vi "microspec_validating - Kopie.vi"() -> ()   [LabVIEW 2013]
uses:
  <vilib>/Instr/_visa.llb/VISA Configure Serial Port (Instr).vi
  <vilib>/Utility/file.llb/Write To Spreadsheet File (string).vi
panel:
  out "error 2":dbl
  in  "Path":path
  in  "intergration time":dbl=54.0 caption="sensor\nintergration time (us)" min=54.0 max=1000000.0 step=100.0
  in  "?":T1(tab)=enum."measuring sequence"
  out "radiometer data file path":path
  in  "Runname":string
  out "Sensor_name":string="ILT1400"
  out "Radiometer Average":dbl
  in  "Delay":dbl=1.0
  in  "Step":dbl=1.0
  in  "Stop Wl":dbl=900.0 min=0.0 max=5000.0 step=100.0
  in  "Start Wl":dbl=300.0 min=0.0 max=5000.0 step=100.0
  in  "mean_number":i32=1 caption="Mean Number"
  out "Current Wavelength":dbl
  out "XY-Graph 2":cluster{"Y":dbl[], "Y":dbl[]}[](graph)
  in  "run 5":bool
  out "sectrometer data file path":path
  in  "save data":bool
  in  "reset with every wavelength?":bool caption="reset with new run?"
  in  "Delay":dbl=1.0
  in  "Step":dbl=10.0
  in  "Stop Wl":dbl=900.0 min=0.0 max=5000.0 step=100.0
  out "Current Wavelength":dbl
  in  "Start Wl 2":dbl=300.0 min=0.0 max=5000.0 step=10.0
  in  "Sensor":string(combo)="C12880MA_15B00040"
  in  "run 2":bool
  in  "Set Runs":i32=1
  out "Current Run":i32
  in  "stop runs":bool
  out "raw_data":cluster{"Y":dbl[], "Y":dbl[]}[](graph) caption="raw data"
  out "error":dbl
  out "raw_data 2":cluster{"Y":dbl[], "Y":dbl[]}[](graph) caption="raw data"
  in  "Stopp":bool
  out "System Setup":i32
  out "DLL Version":string
  out "Get Version":i32
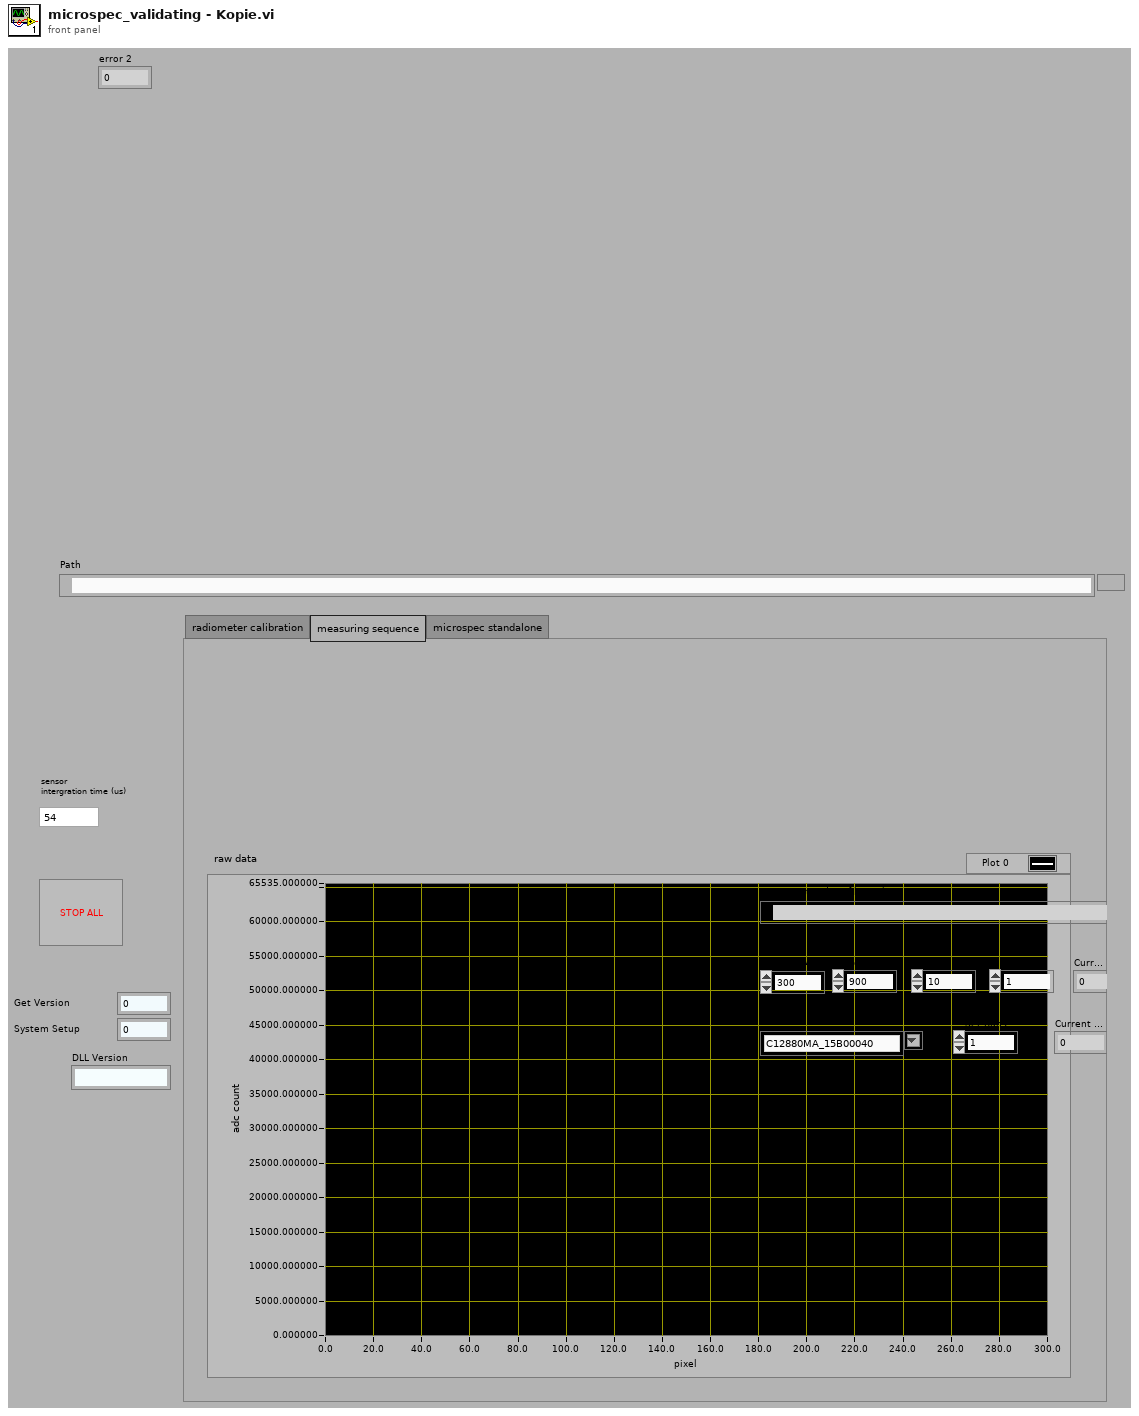
[diagram p1: front panel]
types:
  T1 = enum32{"radiometer calibration", "measuring sequence", "microspec standalone"}
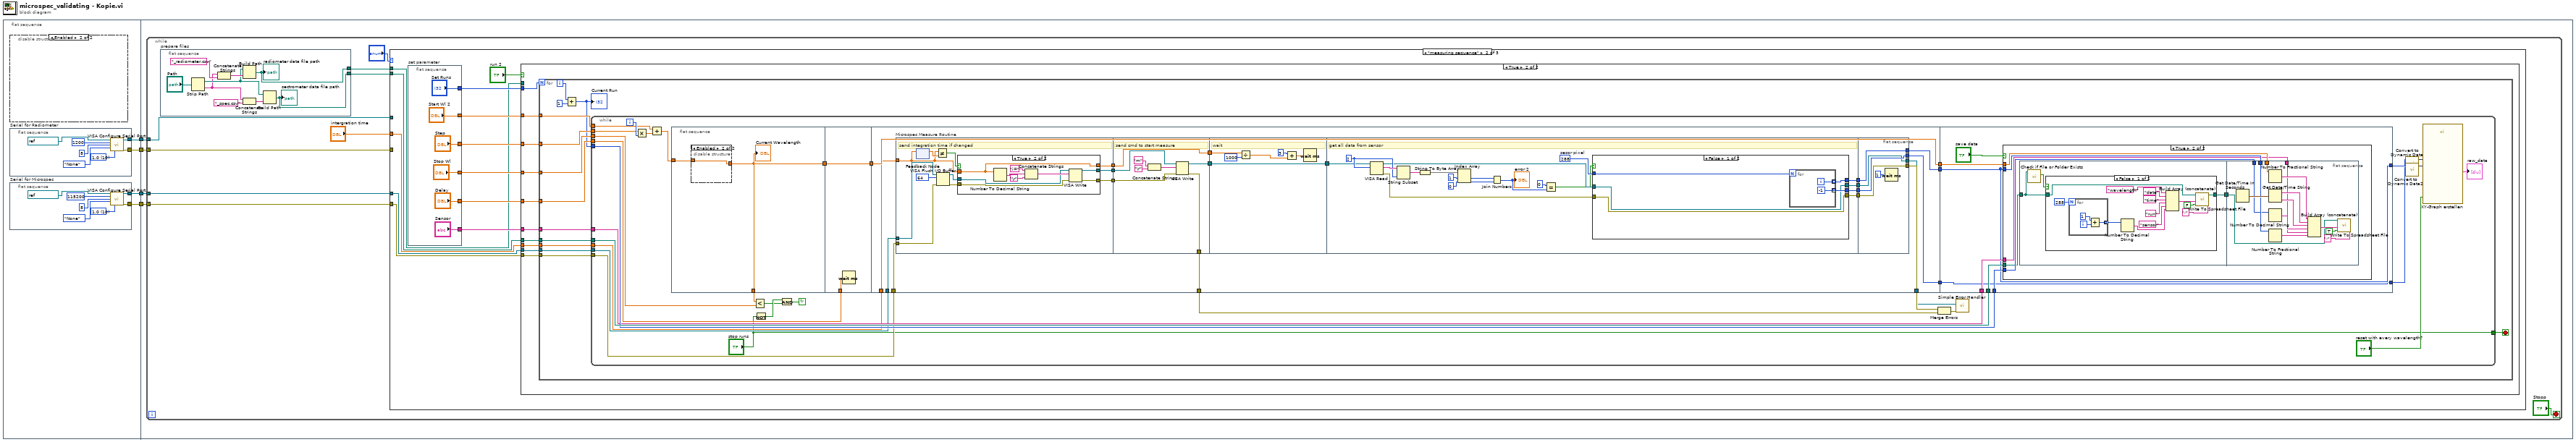
[diagram p0: block diagram]
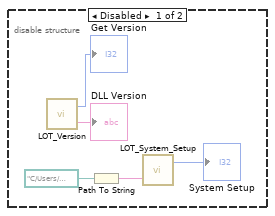
[diagram p2: hidden frame]
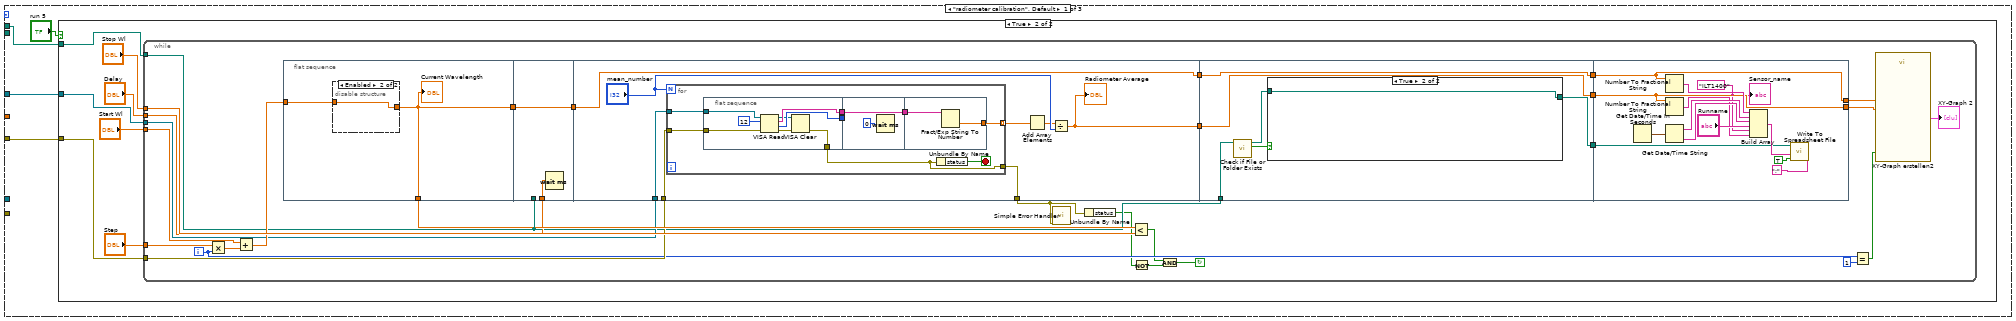
[diagram p3: hidden frame]
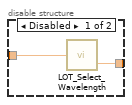
[diagram p5: hidden frame]
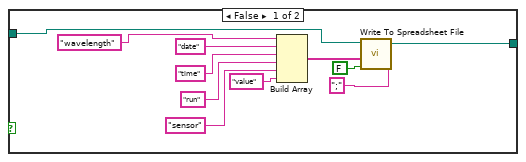
[diagram p6: hidden frame]
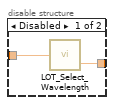
[diagram p8: hidden frame]
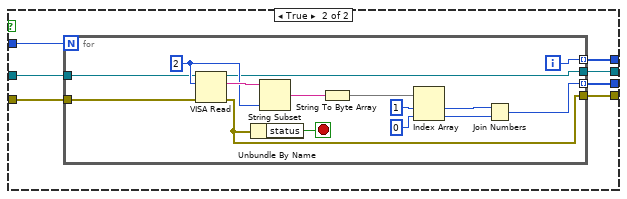
[diagram p10: hidden frame]
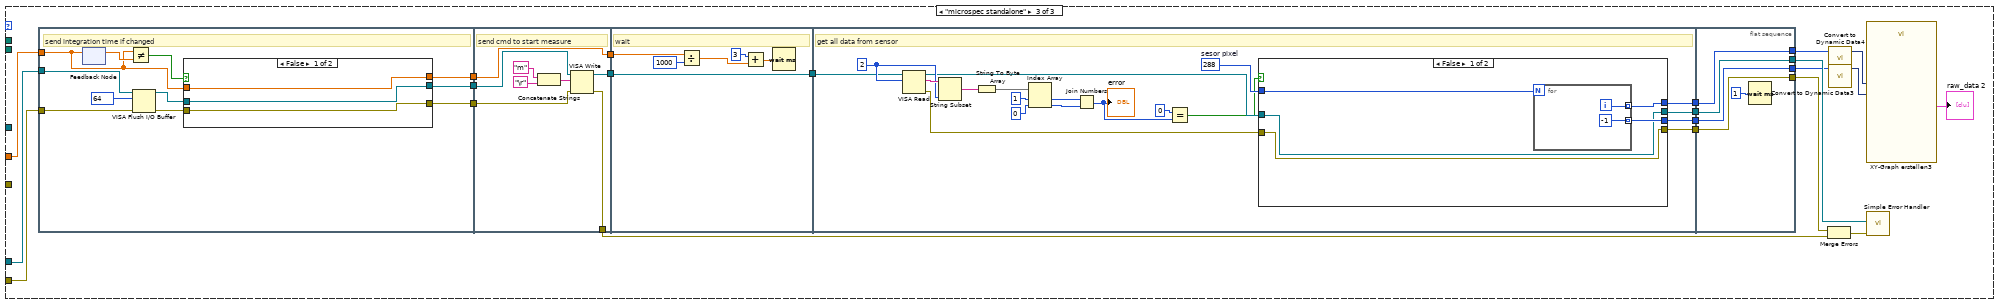
[diagram p13: hidden frame]
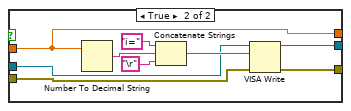
[diagram p14: hidden frame]
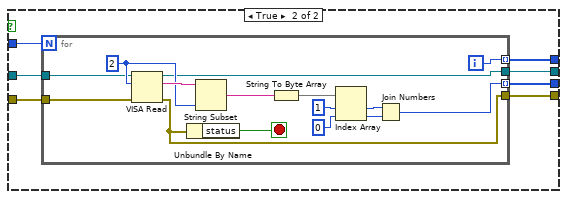
[diagram p15: hidden frame]
diagram:
  n1 = flat-sequence {
    tunnel: [w8] -> w4
    tunnel: [w7] -> w3
    tunnel: [w6] -> w2
    tunnel: [w5] -> w1
    tunnel: w4 -> [w31]
    tunnel: w3 -> [w30]
    tunnel: w2 -> [w29]
    tunnel: w1 -> [w28]
    frame #0 {
      # "Configuration"
      n2 = disable-structure shown="Enabled" {
        frame Disabled {
          n3 = call "LOT_Version.vi"() -> ("Version"=→"DLL Version":string, "Get Version"=→"Get Version":i32)
          n4 = Path To String(path=path "C:/Users/Public/Documents/LOT/Monochromator Control/Configurations/LOT_MSH-300_SN16578.xml" ("Configuration File")) -> (string=w25:string)
          n5 = call "LOT_System_Setup.vi"("CFG File Path"=w25) -> ("Error Code"=→"System Setup":i32)  [unwired: 2 in]
        }
        frame Enabled {
        }
      }
      n6 = flat-sequence "Serial for Radiometer" {
        tunnel: [w15] -> w6
        tunnel: [w14] -> w5
        frame #0 {
          w10 = u16 10 items=["1.0"=10, "1.5"=15, "2.0"=20] ("stop bits (10: 1 bit)")
          n7 = call-poly "VISA Configure Serial Port"("VISA resource name"=refnum<visa-resource-name> "COM4", "baud rate (9600)"=u32 1200, "data bits (8)"=u16 8, "parity (0:none)"=enum16{"None", "Odd", "Even", "Mark", "Space"}."None", "stop bits (10: 1 bit)"=w10) -> ("VISA resource name out"=w14:refnum<visa-resource-name>, "error out"=w15:errorcluster)  [unwired: 9 in]
        }
      }
      n8 = flat-sequence "Serial for Microspec" {
        tunnel: [w22] -> w8
        tunnel: [w21] -> w7
        frame #0 {
          w17 = u16 10 items=["1.0"=10, "1.5"=15, "2.0"=20] ("stop bits (10: 1 bit)")
          n9 = call-poly "VISA Configure Serial Port"("VISA resource name"=refnum<visa-resource-name> "COM11", "baud rate (9600)"=u32 115200, "data bits (8)"=u16 8, "parity (0:none)"=enum16{"None", "Odd", "Even", "Mark", "Space"}."None", "stop bits (10: 1 bit)"=w17) -> ("VISA resource name out"=w22:refnum<visa-resource-name>, "error out"=w21:errorcluster)  [unwired: 9 in]
        }
      }
    }
    frame #1 {
      n10 = while {
        tunnel: w31 -> [w38]
        tunnel: w30 -> [w37]
        tunnel: w29 -> [w36]
        tunnel: w28 -> [w35]
        stop <- "Stopp" stop-if-true
        n11 = flat-sequence "prepare files" {
          tunnel: [w41] -> w32
          tunnel: [w42] -> w33
          frame #0 {
            n12 = Strip Path(path="Path") -> (stripped path=w44:path, name=w43:string)
            n13 = Concatenate Strings(w43, "_radiometer.csv") -> (w45:string)
            n14 = Build Path(base path=w44, name or relative path=w45) -> (appended path=w42:path)
            "radiometer data file path" <- w42
            n15 = Concatenate Strings(w43, "_spec.csv") -> (w47:string)
            n16 = Build Path(base path=w44, name or relative path=w47) -> (appended path=w41:path)
            "sectrometer data file path" <- w41
          }
        }
        n17 = case shown="\"measuring sequence\"" "?" {
          tunnel: w32 -> [_ w165 _]
          tunnel: w38 -> [_ w164 w413]
          tunnel: w37 -> [_ w163 w412]
          tunnel: w36 -> [w52 _ _]
          tunnel: w35 -> [w51 _ _]
          tunnel: "intergration time" -> [_ w162 w411]
          tunnel: w33 -> [w50 w155 _]
          frame "radiometer calibration", Default {
            n18 = case shown="True" "run 5" {
              tunnel: w50 -> [_ w56]
              tunnel: w52 -> [_ w55]
              tunnel: w51 -> [_ w54]
              frame False {
              }
              frame True {
                n19 = while {
                  tunnel: "Step" -> [w88]
                  tunnel: "Start Wl" -> [w86]
                  tunnel: "Stop Wl" -> [w85]
                  tunnel: "Delay" -> [w81]
                  tunnel: w56 -> [w67]
                  tunnel: w54 -> [w80]
                  tunnel: w55 -> [w79]
                  i -> [w75]
                  stop <- w62 continue-if-true
                  n20 = Multiply(x=w88, y=w75) -> (x*y=w87:dbl)
                  n21 = Add(x=w86, y=w87) -> (x+y=w84:dbl)
                  n22 = flat-sequence {
                    tunnel: w84 -> [w90]
                    tunnel: [w89] -> w83
                    tunnel: [w89] -> w82
                    tunnel: w67 -> [_]
                    tunnel: w82 -> [w94]
                    tunnel: w81 -> [w95]
                    tunnel: [w94] -> w78
                    tunnel: w80 -> [w103]
                    tunnel: w79 -> [w102]
                    tunnel: w78 -> [w101]
                    tunnel: [w101] -> w71
                    tunnel: [w99] -> w69
                    tunnel: [w96] -> w61
                    tunnel: w71 -> [w129]
                    tunnel: [w129] -> w70
                    tunnel: w69 -> [w128]
                    tunnel: [w128] -> w68
                    tunnel: w67 -> [w126]
                    tunnel: [w127] -> w66
                    tunnel: [w145] -> w72
                    tunnel: [w146] -> w76
                    tunnel: w70 -> [w146]
                    tunnel: w68 -> [w145]
                    tunnel: w66 -> [w148]
                    frame #0 {
                      n23 = disable-structure shown="Enabled" {
                        disable-tunnel: w90 -> [w92 w93]
                        disable-tunnel: [w91 w93] -> w89
                        frame Disabled {
                          n24 = call "LOT_Select_Wavelength.vi"("Input Wavelength"=w92) -> ("Current Wavelength"=w91:dbl)  [unwired: 1 out]
                        }
                        frame Enabled {
                        }
                      }
                      "Current Wavelength" <- w89
                    }
                    frame #1 {
                      n25 = Wait (ms)(milliseconds to wait=w95) -> ()  [unwired: 1 out]
                    }
                    frame #2 {
                      n26 = for {
                        N: "mean_number" -> [_]
                        tunnel: w103 -> [w108]
                        tunnel: w102 -> [w107]
                        tunnel: [w106] -> w97 mode=indexing
                        tunnel: [w105] -> w96
                        stop <- w104 stop-if-true
                        n27 = flat-sequence {
                          tunnel: [w116] -> w111
                          tunnel: w108 -> [w119]
                          tunnel: w107 -> [w118]
                          tunnel: [w115] -> w110
                          tunnel: [w112] -> w105
                          tunnel: w111 -> [w121]
                          tunnel: [w121] -> w109
                          tunnel: w110 -> [_]
                          tunnel: w109 -> [w122]
                          tunnel: [w123] -> w106
                          frame #0 {
                            n28 = VISA Read(VISA resource name=w119, byte count=12, error in (no error)=w118) -> (VISA resource name out=w113:refnum<visa-resource-name>, read buffer=w116:string, return count=w115:u32, error out=w114:errorcluster)
                            n29 = VISA Clear(VISA resource name=w113, error in (no error)=w114) -> (error out=w112:errorcluster)  [unwired: 1 out]
                          }
                          frame #1 {
                            n30 = Wait (ms)(milliseconds to wait=u32 0 ("Zu wartende ms")) -> ()  [unwired: 1 out]
                          }
                          frame #2 {
                            n31 = Fract/Exp String To Number(string=w122) -> (number=w123:dbl)  [unwired: 3 in, 1 out]
                          }
                        }
                        n32 = Unbundle By Name(w105) -> ("status"=w104:bool)
                      }
                      n33 = Add Array Elements(numeric array=w97) -> (sum=w98:dbl)
                      n34 = Divide(x=w98, y="mean_number") -> (x/y=w99:dbl)
                      "Radiometer Average" <- w99
                    }
                    frame #3 {
                      n35 = call <vilib>:"Check if File or Folder Exists.vi"("path"=w126) -> ("file or folder exists?"=w125:bool, "dup path"=w124:path)  [unwired: 8 in, 1 out]
                      n36 = case shown="True" w125 {
                        tunnel: w124 -> [w138 w141]
                        tunnel: [w131 w141] -> w127
                        frame False {
                          n37 = Build Array("wavelength", "date" ("Element"), "time" ("Element"), "run" ("Element"), "sensor" ("Element"), "value") -> (w140:string[])
                          n38 = call-poly <vilib>:"Write To Spreadsheet File.vi"("delimiter (\\t)"=";", "append to file? (new file:F)"=FALSE, "1D data"=w140, "file path (dialog if empty)"=w138) -> ("new file path (Not A Path if cancelled)"=w131:path)  [unwired: 4 in]
                        }
                        frame True {
                        }
                      }
                    }
                    frame #4 {
                      w143 = "ILT1400" ("Sensor_name")
                      n39 = Get Date/Time In Seconds() -> (seconds since 1Jan1904=w153:timestamp)
                      n40 = Number To Fractional String(number=w146) -> (F-format string=w154:string)  [unwired: 3 in]
                      n41 = Number To Fractional String(number=w145) -> (F-format string=w142:string)  [unwired: 3 in]
                      n42 = Get Date/Time String(seconds (now)=w153) -> (date string=w152:string, time string=w151:string)  [unwired: 2 in]
                      n43 = Build Array(w154, w152, w151, "Runname", w143, w142) -> (w150:string[])
                      n44 = call-poly <vilib>:"Write To Spreadsheet File.vi"("delimiter (\\t)"=";", "append to file? (new file:F)"=TRUE, "1D data"=w150, "file path (dialog if empty)"=w148) -> ()  [unwired: 4 in, 1 out]
                      "Sensor_name" <- w143
                    }
                  }
                  n45 = call <vilib>:"Simple Error Handler.vi"("error in (no error)"=w61) -> ()  [unwired: 4 in, 5 out]
                  n46 = Unbundle By Name(w61) -> ("status"=w63:bool)
                  n47 = Less?(x=w83, y=w85) -> (x < y?=w65:bool)
                  n48 = Not(x=w63) -> (.not. x?=w64:bool)
                  n49 = And(x=w65, y=w64) -> (x .and. y?=w62:bool)
                  n50 = Equal?(x=w75, y=1) -> (x = y?=w73:bool)
                  n51 = call "XY-Graph erstellen2"("Reset"=w73, "Y Input"=w72, "X Input"=w76) -> ("XY Graph"=→"XY-Graph 2":cluster{"Y":dbl[], "Y":dbl[]}[])  [unwired: 7 in, 1 out]
                }
              }
            }
          }
          frame "measuring sequence" {
            n52 = flat-sequence "set parameter" {
              tunnel: ["Sensor"] -> w161
              tunnel: ["Delay"] -> w160
              tunnel: ["Step"] -> w159
              tunnel: ["Stop Wl"] -> w158
              tunnel: ["Start Wl 2"] -> w157
              tunnel: ["Set Runs"] -> w156
              frame #0 {
              }
            }
            n53 = case shown="True" "run 2" {
              tunnel: w165 -> [_ w173]
              tunnel: w161 -> [_ w182]
              tunnel: w156 -> [_ w181]
              tunnel: w164 -> [_ w180]
              tunnel: w163 -> [_ w179]
              tunnel: w160 -> [_ w178]
              tunnel: w158 -> [_ w177]
              tunnel: w159 -> [_ w176]
              tunnel: w157 -> [_ w175]
              tunnel: w162 -> [_ w174]
              tunnel: w155 -> [_ _]
              frame False {
              }
              frame True {
                n54 = for {
                  N: w181 -> [_]
                  tunnel: w173 -> [w195]
                  tunnel: w182 -> [w194]
                  tunnel: w180 -> [w193]
                  tunnel: w179 -> [w192]
                  tunnel: w178 -> [w191]
                  tunnel: w177 -> [w190]
                  tunnel: w176 -> [w189]
                  tunnel: w175 -> [w188]
                  tunnel: w174 -> [w187]
                  i -> [w186]
                  stop <- w183 stop-if-true
                  n55 = Add(x=w186, y=1) -> (x+y=w185:i32)
                  "Current Run" <- w185
                  n56 = while {
                    tunnel: w195 -> [w226]
                    tunnel: w185 -> [w225]
                    tunnel: w194 -> [w221]
                    tunnel: w193 -> [w219]
                    tunnel: w192 -> [w218]
                    tunnel: w191 -> [w209]
                    tunnel: w190 -> [w207]
                    tunnel: w189 -> [w206]
                    tunnel: w188 -> [w205]
                    tunnel: w187 -> [w204]
                    tunnel: ["stop runs"] -> w183
                    i -> [w223]
                    stop <- w198 continue-if-true
                    n57 = Multiply(x=w206, y=w223) -> (x*y=w228:dbl)
                    n58 = Add(x=w205, y=w228) -> (x+y=w227:dbl)
                    n59 = flat-sequence {
                      tunnel: w227 -> [w230]
                      tunnel: [w229] -> w224
                      tunnel: [w229] -> w208
                      tunnel: w224 -> [w234]
                      tunnel: w209 -> [w235]
                      tunnel: [w234] -> w212
                      tunnel: [w243] -> w220
                      tunnel: w219 -> [w247]
                      tunnel: w218 -> [w248]
                      tunnel: [w246] -> w216
                      tunnel: [w245] -> w215
                      tunnel: [w244] -> w214
                      tunnel: w212 -> [w243]
                      tunnel: w204 -> [w242]
                      tunnel: [w241] -> w203
                      tunnel: [w240] -> w196
                      tunnel: w226 -> [w351]
                      tunnel: w220 -> [w350]
                      tunnel: w225 -> [w349]
                      tunnel: [w347] -> w210
                      tunnel: w221 -> [w348]
                      tunnel: w214 -> [w347]
                      tunnel: w203 -> [w346]
                      tunnel: [w346] -> w202
                      frame #0 {
                        # "set wavelength"
                        n60 = disable-structure shown="Enabled" {
                          disable-tunnel: w230 -> [w232 w233]
                          disable-tunnel: [w231 w233] -> w229
                          frame Disabled {
                            n61 = call "LOT_Select_Wavelength.vi"("Input Wavelength"=w232) -> ("Current Wavelength"=w231:dbl)  [unwired: 1 out]
                          }
                          frame Enabled {
                          }
                        }
                        "Current Wavelength" <- w229
                      }
                      frame #1 {
                        # "wait"
                        n62 = Wait (ms)(milliseconds to wait=w235) -> ()  [unwired: 1 out]
                      }
                      frame #2 {
                        n63 = flat-sequence "Microspec Measure Routine" {
                          tunnel: w247 -> [w256]
                          tunnel: w248 -> [w265]
                          tunnel: [w260] -> w254
                          tunnel: [w259] -> w253
                          tunnel: [w258] -> w252
                          tunnel: w242 -> [w255]
                          tunnel: [w282] -> w251
                          tunnel: [w281] -> w245
                          tunnel: w254 -> [w279]
                          tunnel: w253 -> [w280]
                          tunnel: w252 -> [w278]
                          tunnel: [w278] -> w250
                          tunnel: w251 -> [w287]
                          tunnel: [w287] -> w249
                          tunnel: w250 -> [w286]
                          tunnel: w249 -> [w296]
                          tunnel: [w295] -> w239
                          tunnel: [w294] -> w238
                          tunnel: [w293] -> w237
                          tunnel: [w292] -> w236
                          tunnel: [w341] -> w240
                          tunnel: [w342] -> w246
                          tunnel: [w343] -> w241
                          tunnel: [w344] -> w244
                          tunnel: w239 -> [w344]
                          tunnel: w238 -> [w343]
                          tunnel: w237 -> [w342]
                          tunnel: w236 -> [w341]
                          frame #0 {
                            # "send integration time if changed"
                            n64 = feedback #1() -> (w264:dbl)  [unwired: 1 in]
                            n65 = feedback-in #1(w255) -> ()
                            n66 = Not Equal?(x=w255, y=w264) -> (x != y?=w263:bool)
                            n67 = VISA Flush I/O Buffer(VISA resource name=w256, mask (16)=64, error in (no error)=w265) -> (VISA resource name out=w262:refnum<visa-resource-name>, error out=w261:errorcluster)
                            n68 = case shown="True" w263 {
                              tunnel: w262 -> [w267 w273]
                              tunnel: w261 -> [w266 w272]
                              tunnel: [w266 w271] -> w260
                              tunnel: [w267 w270] -> w259
                              tunnel: w255 -> [w268 w269]
                              tunnel: [w268 w269] -> w258
                              frame False {
                              }
                              frame True {
                                n69 = Number To Decimal String(number=w269) -> (decimal integer string=w276:string)  [unwired: 1 in]
                                n70 = Concatenate Strings("i=", w276, "\r") -> (w274:string)
                                n71 = VISA Write(VISA resource name=w273, write buffer=w274, error in (no error)=w272) -> (VISA resource name out=w270:refnum<visa-resource-name>, error out=w271:errorcluster)  [unwired: 1 out]
                              }
                            }
                          }
                          frame #1 {
                            # "send cmd to start measure"
                            n72 = Concatenate Strings("m", "\r") -> (w283:string)
                            n73 = VISA Write(VISA resource name=w280, write buffer=w283, error in (no error)=w279) -> (VISA resource name out=w282:refnum<visa-resource-name>, error out=w281:errorcluster)  [unwired: 1 out]
                          }
                          frame #2 {
                            # "wait"
                            n74 = Divide(x=w286, y=u32 1000 ("Zu wartende ms")) -> (x/y=w288:dbl)
                            n75 = Add(x=u32 3 ("Zu wartende ms"), y=w288) -> (x+y=w290:dbl)
                            n76 = Wait (ms)(milliseconds to wait=w290) -> ()  [unwired: 1 out]
                          }
                          frame #3 {
                            w308 = 2
                            w310 = 288  # sesor pixel
                            # "get all data from sensor"
                            n77 = VISA Read(VISA resource name=w296, byte count=w308) -> (VISA resource name out=w301:refnum<visa-resource-name>, read buffer=w309:string, error out=w298:errorcluster)  [unwired: 1 in, 1 out]
                            n78 = String Subset(string=w309, length (rest)=w308) -> (substring=w307:string)  [unwired: 1 in]
                            n79 = String To Byte Array(string=w307) -> (unsigned byte array=w306:u8[])
                            n80 = Index Array(array=w306, index #1=1, index #2=0) -> (element #1=w302:u8, element #2=w303:u8)
                            n81 = Join Numbers(hi=w302, lo=w303) -> ((hi.lo)=w299:u16)
                            "error 2" <- w299
                            n82 = Equal?(x=0, y=w299) -> (x = y?=w297:bool)
                            n83 = case shown="False" w297 {
                              tunnel: [w313 w324] -> w293
                              tunnel: w301 -> [w312 w323]
                              tunnel: [w314 w322] -> w294
                              tunnel: [w315 w321] -> w295
                              tunnel: w310 -> [w311 w320]
                              tunnel: [w312 w319] -> w292
                              tunnel: w298 -> [w313 w318]
                              frame False {
                                n84 = for {
                                N: w311 -> [_]
                                tunnel: [-1] -> w314 mode=indexing
                                tunnel: [w317] -> w315 mode=indexing
                                i -> [w317]
                                }
                              }
                              frame True {
                                n85 = for {
                                N: w320 -> [_]
                                tunnel: w323 -> [w329]
                                tunnel: [w328] -> w324
                                tunnel: [w331] -> w322 mode=indexing
                                tunnel: [w330] -> w321 mode=indexing
                                tunnel: [w326] -> w319
                                tunnel: w318 -> [w325]
                                i -> [w330]
                                stop <- w327 stop-if-true
                                w338 = 2
                                n86 = VISA Read(VISA resource name=w329, byte count=w338, error in (no error)=w325) -> (VISA resource name out=w326:refnum<visa-resource-name>, read buffer=w339:string, error out=w328:errorcluster)  [unwired: 1 out]
                                n87 = Unbundle By Name(w328) -> ("status"=w327:bool)
                                n88 = String Subset(string=w339, length (rest)=w338) -> (substring=w337:string)  [unwired: 1 in]
                                n89 = String To Byte Array(string=w337) -> (unsigned byte array=w336:u8[])
                                n90 = Index Array(array=w336, index #1=1, index #2=0) -> (element #1=w332:u8, element #2=w333:u8)
                                n91 = Join Numbers(hi=w332, lo=w333) -> ((hi.lo)=w331:u16)
                                }
                              }
                            }
                          }
                          frame #4 {
                            n92 = Wait (ms)(milliseconds to wait=1) -> ()  [unwired: 1 out]
                          }
                        }
                      }
                      frame #3 {
                        n93 = case shown="True" "save data" {
                          tunnel: w351 -> [_ w354]
                          tunnel: w350 -> [_ w356]
                          tunnel: w349 -> [_ w355]
                          tunnel: w347 -> [_ w357]
                          tunnel: w348 -> [_ w353]
                          frame False {
                          }
                          frame True {
                            n94 = flat-sequence {
                              tunnel: w354 -> [w360]
                              tunnel: [w358] -> w352
                              tunnel: w357 -> [w384]
                              tunnel: w356 -> [w383]
                              tunnel: w355 -> [w382]
                              tunnel: w353 -> [w380]
                              tunnel: w352 -> [w378]
                              frame #0 {
                                n95 = call <vilib>:"Check if File or Folder Exists.vi"("path"=w360) -> ("file or folder exists?"=w359:bool)  [unwired: 8 in, 2 out]
                                n96 = case shown="False" w359 {
                                tunnel: w360 -> [w364 w377]
                                tunnel: [w361 w377] -> w358
                                frame False {
                                n97 = for {
                                N: 288 -> [_]
                                tunnel: [w374] -> w367 mode=indexing
                                i -> [w376]
                                n98 = Add(x=1, y=w376) -> (x+y=w374:i32)
                                }
                                n99 = Number To Decimal String(number=w367) -> (decimal integer string=w369:string[])  [unwired: 1 in]
                                n100 = Build Array (concatenate)("wavelength", "date" ("Element"), "time" ("Element"), "run" ("Element"), "sensor" ("Element"), w369) -> (w373:string[])
                                n101 = call-poly <vilib>:"Write To Spreadsheet File.vi"("delimiter (\\t)"=";", "append to file? (new file:F)"=FALSE, "1D data"=w373, "file path (dialog if empty)"=w364) -> ("new file path (Not A Path if cancelled)"=w361:path)  [unwired: 4 in]
                                }
                                frame True {
                                }
                                }
                              }
                              frame #1 {
                                n102 = Get Date/Time In Seconds() -> (seconds since 1Jan1904=w386:timestamp)
                                n103 = Number To Fractional String(number=w383) -> (F-format string=w385:string)  [unwired: 3 in]
                                n104 = Get Date/Time String(seconds (now)=w386) -> (date string=w387:string, time string=w388:string)  [unwired: 2 in]
                                n105 = Number To Decimal String(number=w382) -> (decimal integer string=w381:string)  [unwired: 1 in]
                                n106 = Number To Fractional String(number=w384) -> (F-format string=w391:string[])  [unwired: 3 in]
                                n107 = Build Array (concatenate)(w385, w387, w388, w381, w380, w391) -> (w389:string[])
                                n108 = call-poly <vilib>:"Write To Spreadsheet File.vi"("delimiter (\\t)"=";", "append to file? (new file:F)"=TRUE, "1D data"=w389, "file path (dialog if empty)"=w378) -> ()  [unwired: 4 in, 1 out]
                              }
                            }
                          }
                        }
                      }
                    }
                    n109 = Less?(x=w208, y=w207) -> (x < y?=w199:bool)
                    n110 = Not(x="stop runs") -> (.not. x?=w200:bool)
                    n111 = And(x=w200, y=w199) -> (x .and. y?=w198:bool)
                    n112 = Merge Errors(w216, w215) -> (w217:errorcluster)
                    n113 = call <vilib>:"Simple Error Handler.vi"("error source (\" \")"=w196, "error in (no error)"=w217) -> ()  [unwired: 3 in, 5 out]
                    n114 = call "Convert to Dynamic Data"("Array"=w202) -> ("Dynamic Data Type"=w211:dynamicdata)  [unwired: 3 in]
                    n115 = call "Convert to Dynamic Data2"("Array"=w210) -> ("Dynamic Data Type"=w213:dynamicdata)  [unwired: 3 in]
                    n116 = call "XY-Graph erstellen"("Reset"="reset with every wavelength?", "Y Input"=w213, "X Input"=w211) -> ("XY Graph"=→"raw_data":cluster{"Y":dbl[], "Y":dbl[]}[])  [unwired: 7 in, 1 out]
                  }
                }
              }
            }
          }
          frame "microspec standalone" {
            n117 = flat-sequence {
              tunnel: w413 -> [w423]
              tunnel: w412 -> [w424]
              tunnel: [w418] -> w410
              tunnel: [w417] -> w409
              tunnel: [w416] -> w408
              tunnel: w411 -> [w414]
              tunnel: [w441] -> w407
              tunnel: [w440] -> w403
              tunnel: w410 -> [w438]
              tunnel: w409 -> [w439]
              tunnel: w408 -> [w437]
              tunnel: [w437] -> w406
              tunnel: w407 -> [w446]
              tunnel: [w446] -> w405
              tunnel: w406 -> [w445]
              tunnel: w405 -> [w456]
              tunnel: [w469] -> w395
              tunnel: [w468] -> w394
              tunnel: [w467] -> w393
              tunnel: [w465] -> w392
              tunnel: [w500] -> w401
              tunnel: [w501] -> w396
              tunnel: [w502] -> w397
              tunnel: [w503] -> w404
              tunnel: w395 -> [w503]
              tunnel: w394 -> [w502]
              tunnel: w393 -> [w501]
              tunnel: w392 -> [w500]
              frame #0 {
                # "send integration time if changed"
                n118 = feedback #2() -> (w422:dbl)  [unwired: 1 in]
                n119 = feedback-in #2(w414) -> ()
                n120 = Not Equal?(x=w414, y=w422) -> (x != y?=w421:bool)
                n121 = VISA Flush I/O Buffer(VISA resource name=w423, mask (16)=64, error in (no error)=w424) -> (VISA resource name out=w420:refnum<visa-resource-name>, error out=w419:errorcluster)
                n122 = case shown="False" w421 {
                  tunnel: w420 -> [w426 w432]
                  tunnel: w419 -> [w425 w431]
                  tunnel: [w425 w430] -> w418
                  tunnel: [w426 w429] -> w417
                  tunnel: w414 -> [w427 w428]
                  tunnel: [w427 w428] -> w416
                  frame False {
                  }
                  frame True {
                    n123 = Number To Decimal String(number=w428) -> (decimal integer string=w435:string)  [unwired: 1 in]
                    n124 = Concatenate Strings("i=", w435, "\r") -> (w433:string)
                    n125 = VISA Write(VISA resource name=w432, write buffer=w433, error in (no error)=w431) -> (VISA resource name out=w429:refnum<visa-resource-name>, error out=w430:errorcluster)  [unwired: 1 out]
                  }
                }
              }
              frame #1 {
                # "send cmd to start measure"
                n126 = Concatenate Strings("m", "\r") -> (w442:string)
                n127 = VISA Write(VISA resource name=w439, write buffer=w442, error in (no error)=w438) -> (VISA resource name out=w441:refnum<visa-resource-name>, error out=w440:errorcluster)  [unwired: 1 out]
              }
              frame #2 {
                # "wait"
                n128 = Divide(x=w445, y=u32 1000 ("Zu wartende ms")) -> (x/y=w447:dbl)
                n129 = Add(x=u32 3 ("Zu wartende ms"), y=w447) -> (x+y=w449:dbl)
                n130 = Wait (ms)(milliseconds to wait=w449) -> ()  [unwired: 1 out]
              }
              frame #3 {
                w463 = 2
                w466 = 288  # sesor pixel
                # "get all data from sensor"
                n131 = VISA Read(VISA resource name=w456, byte count=w463) -> (VISA resource name out=w455:refnum<visa-resource-name>, read buffer=w464:string, error out=w452:errorcluster)  [unwired: 1 in, 1 out]
                n132 = String Subset(string=w464, length (rest)=w463) -> (substring=w462:string)  [unwired: 1 in]
                n133 = String To Byte Array(string=w462) -> (unsigned byte array=w461:u8[])
                n134 = Index Array(array=w461, index #1=1, index #2=0) -> (element #1=w457:u8, element #2=w458:u8)
                n135 = Join Numbers(hi=w457, lo=w458) -> ((hi.lo)=w453:u16)
                "error" <- w453
                n136 = Equal?(x=0, y=w453) -> (x = y?=w451:bool)
                n137 = case shown="False" w451 {
                  tunnel: [w472 w483] -> w469
                  tunnel: w455 -> [w471 w482]
                  tunnel: [w473 w481] -> w468
                  tunnel: [w474 w480] -> w467
                  tunnel: w466 -> [w470 w479]
                  tunnel: [w471 w478] -> w465
                  tunnel: w452 -> [w472 w477]
                  frame False {
                    n138 = for {
                      N: w470 -> [_]
                      tunnel: [-1] -> w473 mode=indexing
                      tunnel: [w476] -> w474 mode=indexing
                      i -> [w476]
                    }
                  }
                  frame True {
                    n139 = for {
                      N: w479 -> [_]
                      tunnel: w482 -> [w488]
                      tunnel: [w487] -> w483
                      tunnel: [w490] -> w481 mode=indexing
                      tunnel: [w489] -> w480 mode=indexing
                      tunnel: [w485] -> w478
                      tunnel: w477 -> [w484]
                      i -> [w489]
                      stop <- w486 stop-if-true
                      w497 = 2
                      n140 = VISA Read(VISA resource name=w488, byte count=w497, error in (no error)=w484) -> (VISA resource name out=w485:refnum<visa-resource-name>, read buffer=w498:string, error out=w487:errorcluster)  [unwired: 1 out]
                      n141 = Unbundle By Name(w487) -> ("status"=w486:bool)
                      n142 = String Subset(string=w498, length (rest)=w497) -> (substring=w496:string)  [unwired: 1 in]
                      n143 = String To Byte Array(string=w496) -> (unsigned byte array=w495:u8[])
                      n144 = Index Array(array=w495, index #1=1, index #2=0) -> (element #1=w491:u8, element #2=w492:u8)
                      n145 = Join Numbers(hi=w491, lo=w492) -> ((hi.lo)=w490:u16)
                    }
                  }
                }
              }
              frame #4 {
                n146 = Wait (ms)(milliseconds to wait=1) -> ()  [unwired: 1 out]
              }
            }
            n147 = Merge Errors(w404, w403) -> (w402:errorcluster)
            n148 = call "Convert to Dynamic Data4"("Array"=w396) -> ("Dynamic Data Type"=w398:dynamicdata)  [unwired: 3 in]
            n149 = call "Convert to Dynamic Data3"("Array"=w397) -> ("Dynamic Data Type"=w399:dynamicdata)  [unwired: 3 in]
            n150 = call "XY-Graph erstellen3"("Y Input"=w399, "X Input"=w398) -> ("XY Graph"=→"raw_data 2":cluster{"Y":dbl[], "Y":dbl[]}[])  [unwired: 8 in, 1 out]
            n151 = call <vilib>:"Simple Error Handler.vi"("error source (\" \")"=w401, "error in (no error)"=w402) -> ()  [unwired: 3 in, 5 out]
          }
        }
      }
    }
  }
